vi "102-3102-report4part2-gaydos.vi"() -> ()   [LabVIEW 2011]
uses:
  <vilib>/imath/engines/lvmath2/RunTimeEngine/ErrorHandling/NIMS_Finalize Error.vi
  <vilib>/imath/engines/lvmath2/RunTimeEngine/Managers/WorkSpace/UID Generator.vi
  <vilib>/imath/engines/lvmath2/RunTimeEngine/NodeEndStatement/NIMS_NodeEndStatement_Get Vector.vi
  <instcachedir>/0/NIMS_NodeEndStatement_Get Vector_50E2F48DC826428EA11CD85545CBACBE.lvgen/NIMS_NodeEndStatement_Get Vector_50E2F48DC826428EA11CD85545CBACBE_001.vi
  <vilib>/imath/engines/lvmath/Functions/Error Handling/MergeErrorsWrapper.vi
  <vilib>/imath/engines/lvmath2/RunTimeEngine/Managers/SymbolTable/Clear UID.vi
  <vilib>/imath/engines/lvmath2/RunTimeEngine/NodeEndStatement/NIMS_NodeEndStatement_Output.vi
  <instcachedir>/0/NIMS_NodeEndStatement_Output_53EC0D466D134D7ABD903AC30B43404B.lvgen/NIMS_NodeEndStatement_Output_53EC0D466D134D7ABD903AC30B43404B_005.vi
  <instcachedir>/0/NIMS_NodeEndStatement_Output_53EC0D466D134D7ABD903AC30B43404B.lvgen/NIMS_NodeEndStatement_Output_53EC0D466D134D7ABD903AC30B43404B_001.vi
  <vilib>/imath/engines/lvmath2/RunTimeEngine/RangeToken/NIMS_Range.vi
  <instcachedir>/0/NIMS_Range_0B7635FB69F84E19AA68E7FF959DF37C.lvgen/NIMS_Range_0B7635FB69F84E19AA68E7FF959DF37C_001.vi
  <vilib>/imathl/engines/lvmath/Functions/Error Handling/Create Error.vi
  <vilib>/imath/engines/lvmath2/RunTimeEngine/BuiltInFunctions/zeros/NIMS_V=zeros(I32,I32).vi
  <vilib>/imath/engines/lvmath2/RunTimeEngine/RunTimeType/NIMS_RunTimeType_From StrictType (excl LVString).vi
  <instcachedir>/0/NIMS_RunTimeType_From StrictType (excl LVString)_46AE8B54A11948F0BCCEB8091EE7AA4C.lvgen/NIMS_RunTimeType_From StrictType (excl LVString)_46AE8B54A11948F0BCCEB8091EE7AA4C_000.vi
  <vilib>/imath/engines/lvmath2/RunTimeEngine/LocalVariableDefStatement/MC_LocalVariableDefStatement_Display.vi
  <vilib>/imath/engines/lvmath2/RunTimeEngine/BuiltInFunctions/repeatmx/NIMS_repeatmx(GM, I32, I32).vi
  <instcachedir>/0/NIMS_repeatmx(GM, I32, I32)_8C2ED2EBCBCE41FC8E83AC0E124C0986.lvgen/NIMS_repeatmx(GM, I32, I32)_8C2ED2EBCBCE41FC8E83AC0E124C0986_000.vi
  <vilib>/imath/engines/lvmath2/RunTimeEngine/BuiltInFunctions/length/NIMS_length(GV).vi
  <instcachedir>/0/NIMS_length(GV)_08A3D13377FD4E4B96F5795FBF3698FA.lvgen/NIMS_length(GV)_08A3D13377FD4E4B96F5795FBF3698FA_000.vi
  <vilib>/imath/engines/lvmath2/RunTimeEngine/BuiltInFunctions/mean/NIMS_RS=mean(RV,I32).vi
  <vilib>/imath/engines/lvmath2/RunTimeEngine/RangeToken/NIMS_Range_R2 - Float.vi
  <instcachedir>/0/NIMS_Range_R2 - Float_C1282E71A4144327AAA2CE46E2A27C60.lvgen/NIMS_Range_R2 - Float_C1282E71A4144327AAA2CE46E2A27C60_000.vi
  <vilib>/imath/engines/lvmath2/RunTimeEngine/CommandStatement/MC_CommandStatement_break.vi
  <instcachedir>/0/NIMS_Range_0B7635FB69F84E19AA68E7FF959DF37C.lvgen/NIMS_Range_0B7635FB69F84E19AA68E7FF959DF37C_000.vi
  <vilib>/imath/engines/lvmath2/RunTimeEngine/VariableToken/NIMS_VariableToken_CondDefinedDefinedByReplace.vi
  <instcachedir>/0/NIMS_VariableToken_CondDefinedDefinedByReplace_D162CFFC24174562A9FEA619A91E1A56.lvgen/NIMS_VariableToken_CondDefinedDefinedByReplace_D162CFFC24174562A9FEA619A91E1A56_002.vi
  <vilib>/imath/engines/lvmath2/RunTimeEngine/ReplaceToken/NIMS_Replace - Check(_) Linear.vi
  <instcachedir>/0/NIMS_Replace - Check(_) Linear_271D1740B3B04FAC84D127F9D4901600.lvgen/NIMS_Replace - Check(_) Linear_271D1740B3B04FAC84D127F9D4901600_008.vi
  <vilib>/imath/engines/lvmath2/RunTimeEngine/ArithmeticOperatorToken/NIMS_ArithmeticOperator_times.vi
  <instcachedir>/0/NIMS_ArithmeticOperator_times_3FA9DDB491BD45F6905798C0465C9825.lvgen/NIMS_ArithmeticOperator_times_3FA9DDB491BD45F6905798C0465C9825_000.vi
  <vilib>/imath/engines/lvmath2/RunTimeEngine/BuiltInFunctions/sum/NIMS_sum(GV).vi
  <instcachedir>/0/NIMS_sum(GV)_67F5EC36BC034E54A6BEC5B0673C00E5.lvgen/NIMS_sum(GV)_67F5EC36BC034E54A6BEC5B0673C00E5_000.vi
  <vilib>/imath/engines/lvmath2/RunTimeEngine/ReplaceToken/NIMS_Replace - Size Check _(_)=S.vi
  <instcachedir>/0/NIMS_Replace - Size Check _(_)=S_9ABE7AF2D26C43EAA05192D5C1E6C624.lvgen/NIMS_Replace - Size Check _(_)=S_9ABE7AF2D26C43EAA05192D5C1E6C624_000.vi
  <vilib>/imath/engines/lvmath2/RunTimeEngine/ReplaceToken/NIMS_Replace - V(S)=S.vi
  <instcachedir>/0/NIMS_Replace - V(S)=S_16B13A4565AB46F59881314645612498.lvgen/NIMS_Replace - V(S)=S_16B13A4565AB46F59881314645612498_000.vi
  <vilib>/imath/engines/lvmath2/RunTimeEngine/ErrorHandling/NIMS_Create Error From Enums.vi
  <vilib>/imath/engines/lvmath2/RunTimeEngine/BuiltInFunctions/length/NIMS_length(GM).vi
  <instcachedir>/0/NIMS_length(GM)_47CEC356FCE0482D9BA47DC61C99F2C7.lvgen/NIMS_length(GM)_47CEC356FCE0482D9BA47DC61C99F2C7_000.vi
  <vilib>/imath/engines/lvmath2/RunTimeEngine/BuiltInFunctions/ones/NIMS_V=ones(I32,I32).vi
  <vilib>/imath/engines/lvmath2/RunTimeEngine/VariableToken/NIMS_VariableToken_CondDefined.vi
  <instcachedir>/0/NIMS_VariableToken_CondDefined_D30D2F4D3CE04567BC79CC35D27951F7.lvgen/NIMS_VariableToken_CondDefined_D30D2F4D3CE04567BC79CC35D27951F7_003.vi
  <vilib>/imath/engines/lvmath2/RunTimeEngine/VariableToken/Read/NIMS_Get Elements - RV(_) - Check(_).vi
  <instcachedir>/0/NIMS_Get Elements - RV(_) - Check(_)_95E78A4FFA0646428F3543E57837F638.lvgen/NIMS_Get Elements - RV(_) - Check(_)_95E78A4FFA0646428F3543E57837F638_000.vi
  <vilib>/imath/engines/lvmath2/RunTimeEngine/ArithmeticOperatorToken/NIMS_ArithmeticOperator_plus.vi
  <instcachedir>/0/NIMS_ArithmeticOperator_plus_1E95F7DAB906458CBECCADBE8E6FD739.lvgen/NIMS_ArithmeticOperator_plus_1E95F7DAB906458CBECCADBE8E6FD739_004.vi
  <vilib>/imath/engines/lvmath2/RunTimeEngine/ArithmeticOperatorToken/NIMS_ArithmeticOperator_minus.vi
  <instcachedir>/0/NIMS_ArithmeticOperator_minus_27860A2576AF4B729B9D72749D8AAD88.lvgen/NIMS_ArithmeticOperator_minus_27860A2576AF4B729B9D72749D8AAD88_003.vi
  <instcachedir>/0/NIMS_ArithmeticOperator_minus_27860A2576AF4B729B9D72749D8AAD88.lvgen/NIMS_ArithmeticOperator_minus_27860A2576AF4B729B9D72749D8AAD88_002.vi
  <vilib>/imath/engines/lvmath2/RunTimeEngine/BuiltInFunctions/abs/NIMS_abs(signed).vi
  <instcachedir>/0/NIMS_abs(signed)_C4FCB8E6058B49B797C7C8D53CA5F6EC.lvgen/NIMS_abs(signed)_C4FCB8E6058B49B797C7C8D53CA5F6EC_005.vi
  <vilib>/imath/engines/lvmath2/RunTimeEngine/BuiltInFunctions/max/1 input/NIMS_max(RM).vi
  <instcachedir>/0/NIMS_max(RM)_D1651FFEDB2B4E4A81A1820145941633.lvgen/NIMS_max(RM)_D1651FFEDB2B4E4A81A1820145941633_000.vi
  <vilib>/imath/engines/lvmath2/RunTimeEngine/Managers/SymbolTable/NIMS_WorkSpace.lvlib
panel:
  out "yhatz":waveform(dbl)(graph)
  out "xhatz":waveform(dbl)(graph)
  out "Waveform Graph":waveform(dbl)(graph)
  in  "N":dbl
  in  "T":dbl
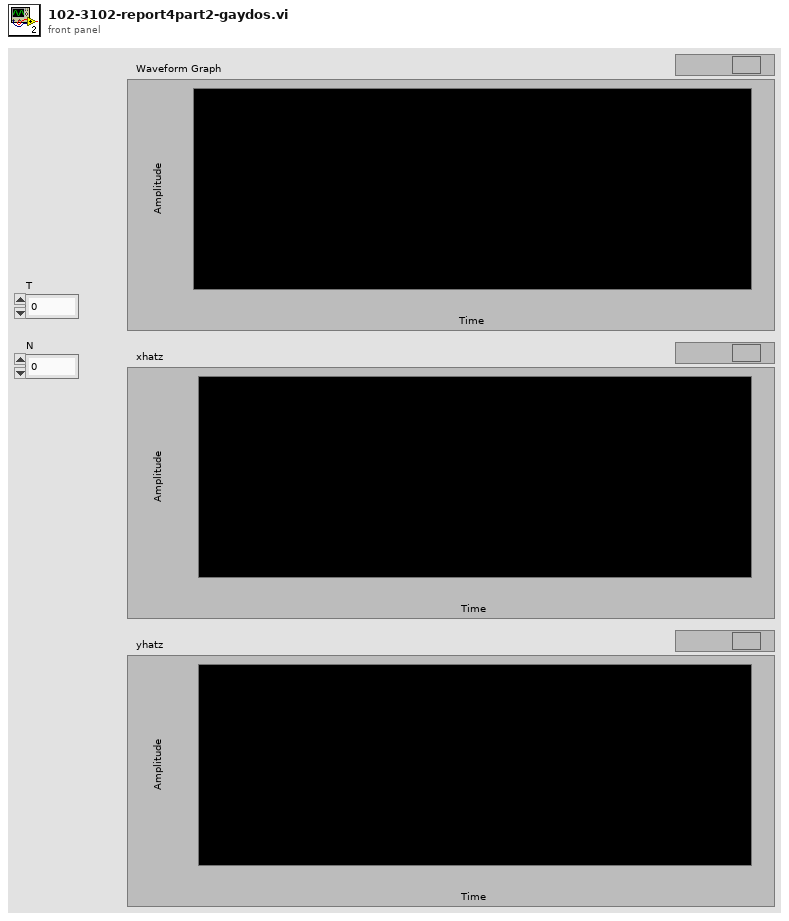
[diagram p1: front panel]
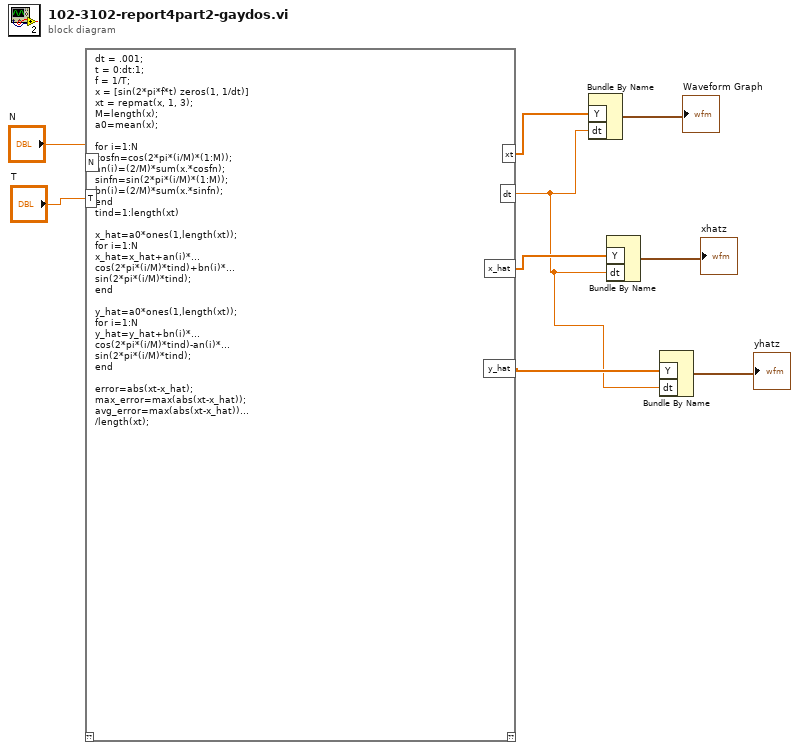
[diagram p0: block diagram]
diagram:
  n1 = mathscript code="dt = .001;\nt = 0:dt:1;\nf = 1/T;\nx = [sin(2*pi*f*t) zeros(1, 1/dt)]\nxt = repmat(x, 1, 3);\nM=length(x);\na0=mean(x);\n\nfor i=1:N\ncosfn=cos(2*pi*(i/M)*(1:M));\nan(i)=(2/M)*sum(x.*cosfn);\nsinfn=sin(2*pi*(i/M)*(1:M));\nbn(i)=(2/M)*sum(x.*sinfn);\nend\ntind=1:length(xt)\n\nx_hat=a0*ones(1,length(xt));\nfor i=1:N\nx_hat=x_hat+an(i)*...\ncos(2*pi*(i/M)*tind)+bn(i)*...\nsin(2*pi*(i/M)*tind);\nend\n\ny_hat=a0*ones(1,length(xt));\nfor i=1:N\ny_hat=y_hat+bn(i)*...\ncos(2*pi*(i/M)*tind)-an(i)*...\nsin(2*pi*(i/M)*tind);\nend\n\nerror=abs(xt-x_hat);\nmax_error=max(abs(xt-x_hat));\navg_error=max(abs(xt-x_hat))...\n/length(xt);"("N"="N", "T"="T") -> ("xt"=w7:dbl[], "dt"=w1:dbl, "x_hat"=w4:dbl[], "y_hat"=w2:dbl[])  [unwired: 1 in, 1 out]
  n2 = Bundle By Name("Y"=w7, "dt"=w1) -> (→"Waveform Graph":waveform(dbl))  [unwired: 1 in]
  n3 = Bundle By Name("Y"=w4, "dt"=w1) -> (→"xhatz":waveform(dbl))  [unwired: 1 in]
  n4 = Bundle By Name("Y"=w2, "dt"=w1) -> (→"yhatz":waveform(dbl))  [unwired: 1 in]
